vi "PathPlanner_CommandUtil_DoStartStop.vi"(9 "Enter_Exit":bool, 11 "Event Action Name":string) -> ()   [LabVIEW 2019, in "PathPlanner24.lvlib"]
uses:
  PathPlanner24.lvlib
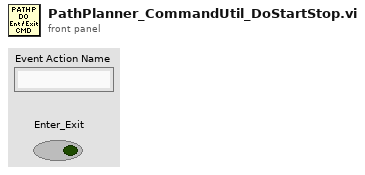
[diagram p1: front panel]
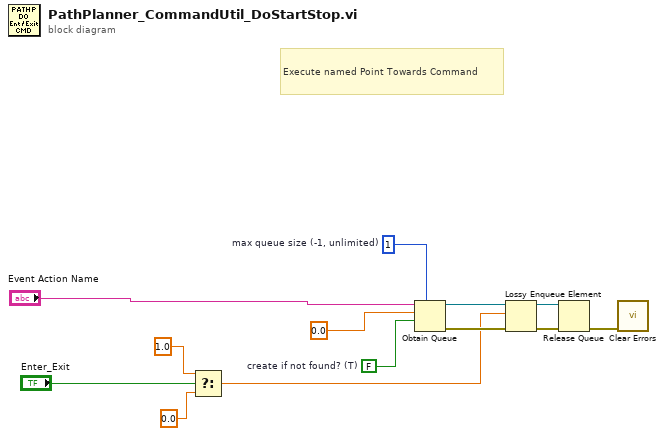
[diagram p0: block diagram]
diagram:
  w12 = FALSE  # create if not found? (T)
  w13 = 1  # max queue size (-1, unlimited)
  # "Execute named Point Towards Command"
  n1 = Select(t=1.0, s="Enter_Exit", f=0.0) -> (s? t:f=w4:dbl)
  n2 = Obtain Queue(max queue size (-1, unlimited)=w13, name (unnamed)="Event Action Name", element data type=0.0, create if not found? (T)=w12) -> (queue out=w9:refnum<queue>, error out=w8:errorcluster)  [unwired: 1 in, 1 out]
  n3 = Lossy Enqueue Element(queue=w9, element=w4, error in (no error)=w8) -> (queue out=w2:refnum<queue>, error out=w1:errorcluster)  [unwired: 2 out]
  n4 = Release Queue(queue=w2, error in (no error)=w1) -> (error out=w3:errorcluster)  [unwired: 1 in, 2 out]
  n5 = call <vilib>:"Clear Errors.vi"("error in (no error)"=w3) -> ()  [unwired: 5 in, 2 out]
